vi "GPS_HeadingChangeEventExe.vi"(0 "Devices In":u64[](array[numeric]), 5 "Event Registration Refnum In":refnum<event-registration>, 11 "error in (no error)":errorcluster) -> (1 "Index":i32, 3 "Event?":bool, 4 "Devices Out":u64[](array[numeric]), 6 "Event Registration Refnum Out":refnum<event-registration>, 8 "Heading":dbl, 10 "Velocity":dbl, 14 "phid":u64, 15 "error out":errorcluster)   [LabVIEW 2012, in "Phidget GPS.lvlib"]
doc: "${HeadingChange:Header}"
uses:
  <instrlib>/Phidgets/Phidget GPS/Phidget GPS.lvlib
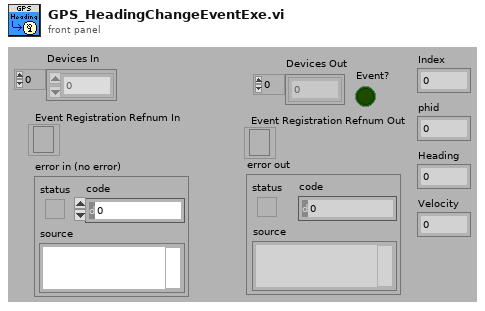
[diagram p1: front panel]
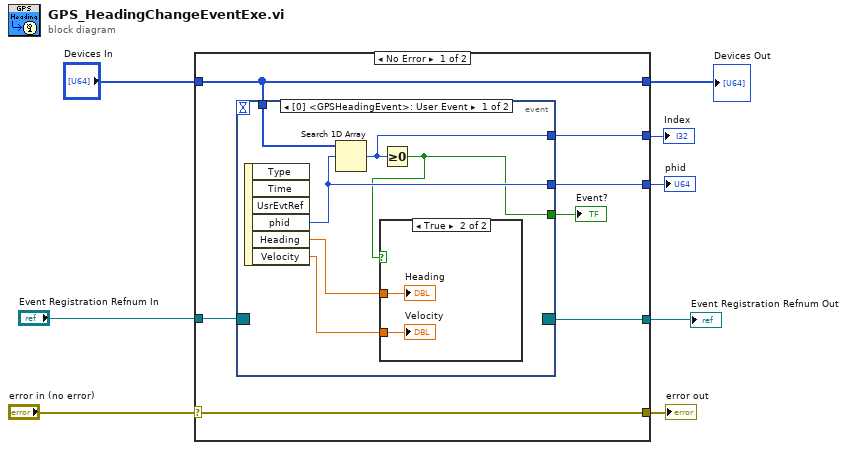
[diagram p0: block diagram]
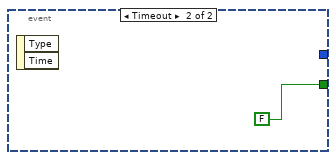
[diagram p3: hidden frame]
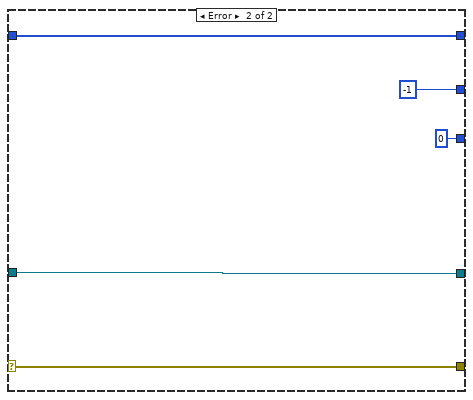
[diagram p4: hidden frame]
diagram:
  n1 = case shown="No Error" "error in (no error)" {
    selector: "error in (no error)" -> [w13 w29]
    tunnel: [w13 w29] -> w7
    tunnel: [w15 w28] -> w1
    tunnel: "Event Registration Refnum In" -> [w14 w28]
    tunnel: [w12 w27] -> w5
    tunnel: "Devices In" -> [w12 w27]
    tunnel: [w11 -1] -> w4
    tunnel: [w10 u64 0 ("phid")] -> w3
    frame No Error {
      n2 = event shown="[0] <GPSHeadingEvent>: User Event" {
        selector: w14 -> [_ _]
        dyn-events: [_ _] -> w15
        timeout: _ -> [_ _]
        tunnel: w12 -> [w21 _]
        tunnel: [w20 _] -> w11
        tunnel: [w18 _] -> w10
        tunnel: [w17 FALSE] -> w9
        event User Event {
          n3 = event-data() -> ("phid"=w18:u64, "Heading"=w19:dbl, "Velocity"=w16:dbl)  [unwired: 1 in, 3 out]
          n4 = Search 1D Array(1D array=w21, element=w18) -> (index of element=w20:i32)  [unwired: 1 in]
          n5 = Greater Or Equal To 0?(x=w20) -> (x >= 0?=w17:bool)
          n6 = case shown="True" w17 {
            tunnel: w19 -> [_ w23]
            tunnel: w16 -> [_ w22]
            frame False {
            }
            frame True {
              "Heading" <- w23
              "Velocity" <- w22
            }
          }
        }
        event Timeout {
          n7 = event-data() -> ()  [unwired: 1 in, 2 out]
        }
      }
      "Event?" <- w9
    }
    frame Error {
    }
  }
  "error out" <- w7
  "Devices Out" <- w5
  "Index" <- w4
  "phid" <- w3
  "Event Registration Refnum Out" <- w1
